vi "Template - Spectrum Analyzer Acquire Trace.vi"() -> ()   [LabVIEW 2013]
doc: "This example shows how to configure the spectrum analyzer to acquire a trace."
uses:
  <instrlib>/_Template - Spectrum Analyzer/Public/Configure/Configure Frequency (Start Stop).vi
  <instrlib>/_Template - Spectrum Analyzer/Template - Spectrum Analyzer.lvlib
panel:
  out "Trace Waveform":T1(graph)
  in  "Manual Detector Type (0: Positive)":u16(ring) items=["Positive", "RMS", "Negative", "Sample"]
  in  "Reference Level Offset (0 dB)":dbl
  in  "Reference Level (10 dBm)":dbl=10.0
  in  "Input Impedance (0: 50 ohms)":u16(ring) items=["50", "75"]
  in  "Trace Type (0: Clear Write)":u16(ring) items=["Clear Write", "Maximum Hold", "Minimum Hold", "View"]
  in  "Stop Frequency (2 GHz)":dbl=2000000000.0
  in  "Start Frequency (0 Hz)":dbl
  in  "VISA resource name":refnum<visa-resource-name>
  # "(c) 2007 <Enter Company Name Here>.  ALL RIGHTS RESERVED."
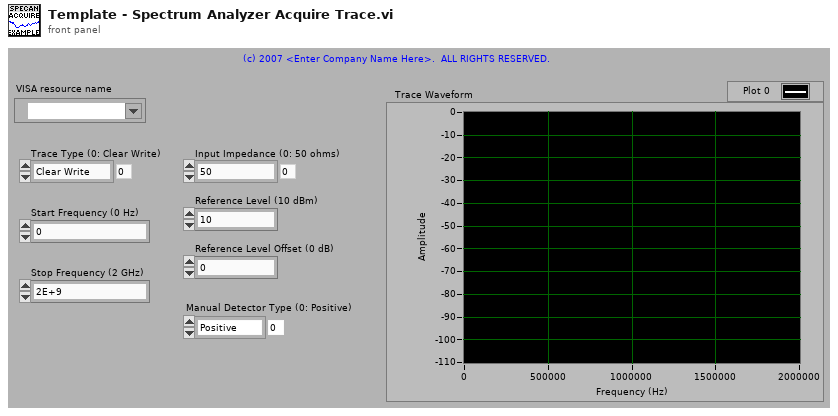
[diagram p1: front panel]
types:
  T1 = cluster{"Start Frequency (0 Hz)":dbl, dbl, "Trace":sgl[]}
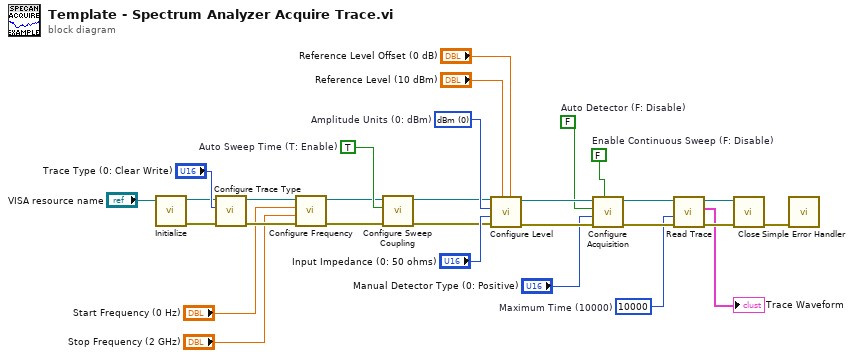
[diagram p0: block diagram]
diagram:
  w1 = u32 10000  # Maximum Time (10000)
  w10 = TRUE  # Auto Sweep Time (T: Enable)
  w16 = FALSE  # Auto Detector (F: Disable)
  w17 = FALSE  # Enable Continuous Sweep (F: Disable)
  w21 = u16 0 items=["dBm", "dBV", "dBmV", "dBuV", "Volts", "Watts"]  # Amplitude Units (0: dBm)
  n1 = call <instrlib>:"Initialize.vi"("VISA resource name"="VISA resource name") -> ("error out"=w13:errorcluster, "VISA resource name out"=w14:refnum<visa-resource-name>)  [unwired: 9 in]
  n2 = call <instrlib>:"Configure Trace Type.vi"("error in (no error)"=w13, "Trace Type (0: Clear Write)"="Trace Type (0: Clear Write)", "VISA resource name"=w14) -> ("error out"=w4:errorcluster, "VISA resource name out"=w7:refnum<visa-resource-name>)  [unwired: 7 in]
  n3 = call-poly <instrlib>:"Configure Frequency.vi"("error in (no error)"=w4, "Stop Frequency (2 GHz)"="Stop Frequency (2 GHz)", "Start Frequency (0 Hz)"="Start Frequency (0 Hz)", "VISA resource name"=w7) -> ("error out"=w5:errorcluster, "VISA resource name out"=w6:refnum<visa-resource-name>)  [unwired: 6 in]
  n4 = call <instrlib>:"Configure Sweep Coupling.vi"("error in (no error)"=w5, "Auto Sweep Time (T: Enable)"=w10, "VISA resource name"=w6) -> ("error out"=w11:errorcluster, "VISA resource name out"=w12:refnum<visa-resource-name>)  [unwired: 7 in]
  n5 = call <instrlib>:"Configure Level.vi"("Reference Level Offset (0 dB)"="Reference Level Offset (0 dB)", "Reference Level (0)"="Reference Level (10 dBm)", "error in (no error)"=w11, "Input Impedance (0: 50 ohms)"="Input Impedance (0: 50 ohms)", "Amplitude Units (0: dBm)"=w21, "VISA resource name"=w12) -> ("error out"=w22:errorcluster, "VISA resource name out"=w23:refnum<visa-resource-name>)  [unwired: 4 in]
  n6 = call <instrlib>:"Configure Acquisition.vi"("Enable Continuous Sweep (F: Disable)"=w17, "error in (no error)"=w22, "Manual Detector Type (0: Positive)"="Manual Detector Type (0: Positive)", "Auto Detector (F: Disable)"=w16, "VISA resource name"=w23) -> ("error out"=w29:errorcluster, "VISA resource name out"=w28:refnum<visa-resource-name>)  [unwired: 5 in]
  n7 = call <instrlib>:"Read Trace.vi"("error in (no error)"=w29, "Maximum Time (10000)"=w1, "VISA resource name"=w28) -> ("error out"=w25:errorcluster, "Trace Waveform"=→"Trace Waveform":T1, "VISA resource name out"=w27:refnum<visa-resource-name>)  [unwired: 6 in]
  n8 = call <instrlib>:"Close.vi"("error in (no error)"=w25, "VISA resource name"=w27) -> ("error out"=w26:errorcluster)  [unwired: 9 in]
  n9 = call <vilib>:"Simple Error Handler.vi"("error in (no error)"=w26) -> ()  [unwired: 4 in, 5 out]
